vi "Mask Write Holding Register.vi"(5 "OR mask":u16, 7 "AND mask":u16, 8 "error in (no error)":errorcluster, 10 "address":u16, 11 "MB session in":refnum<class "MB_Master.lvclass">) -> (0 "error out":errorcluster, 3 "MB session out":refnum<class "MB_Master.lvclass">)   [LabVIEW 2023, in "MB Master.lvlib"]
doc: "Function Code 22: Modifies value of holding register at <b>address</b> based on the <b>AND mask</b> and <b>OR mask</b>.\n\nThe slave device implements the following formula to modify the register's value:\nResult = (Current Value AND And_Mask) OR (Or_Mask AND (NOT And_Mask))\n\nSet bits to 0 in AND mask to specify which bits to modify. Use OR mask to specify the value of bits.\n\nExample:\nRegister Value: 1100 0001\nAND Mask: 1111 1100\nOR Mask: 0000 0010\nResult: 1100 0010"
uses:
  <vilib>/Plasmionique/MB Master/MB Master.lvlib
  <vilib>/Plasmionique/MB Master/MB_Master/MB_Master.lvclass
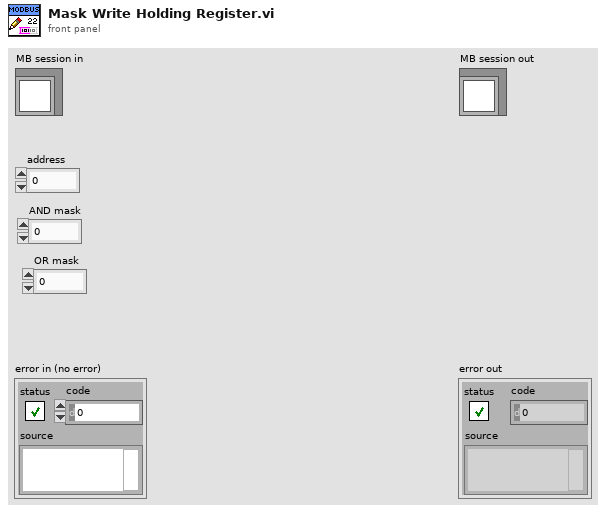
[diagram p1: front panel]
types:
  T1 = typedef "MB Master.lvlib/MB_PDU_Cluster.ctl" = cluster{"Function Code":u8, "Data":u8[], "RTU_DataBytes":i32}
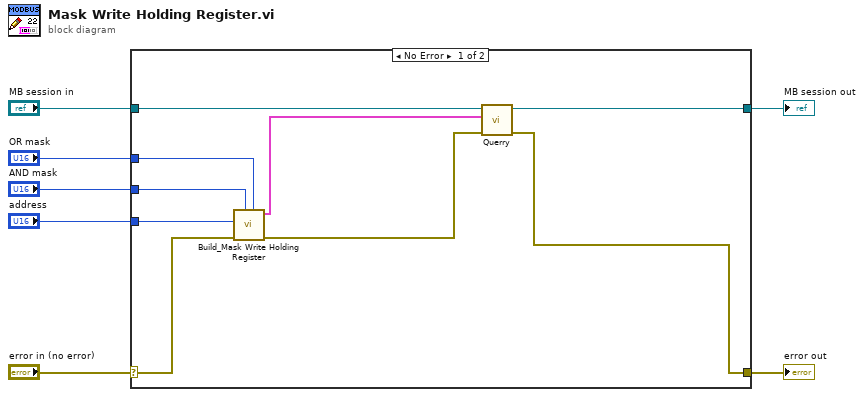
[diagram p0: block diagram]
diagram:
  n1 = case shown="No Error" "error in (no error)" {
    selector: "error in (no error)" -> [w12 w18]
    tunnel: [w15 w18] -> w6
    tunnel: [w16 w17] -> w4
    tunnel: "MB session in" -> [w14 w17]
    tunnel: "address" -> [w11 _]
    tunnel: "AND mask" -> [w10 _]
    tunnel: "OR mask" -> [w9 _]
    frame No Error {
      n2 = call <vilib>:"Build_Mask Write Holding Register.vi"("OR mask"=w9, "AND mask"=w10, "error in (no error)"=w12, "starting address"=w11) -> ("error out"=w13:errorcluster, "MB_PDU"=w8:T1)  [unwired: 6 in]
      n3 = call-dynamic "Querry.vi"("error in (no error)"=w13, "PDU_req"=w8, "MB_Master in"=w14) -> ("error out"=w15:errorcluster, "MB_Master out"=w16:refnum<class "MB_Master.lvclass">)  [unwired: 6 in, 1 out]
    }
    frame Error {
    }
  }
  "error out" <- w6
  "MB session out" <- w4
